vi "disconnect and destroy.vi"(8 "error in (no error)":errorcluster, 11 "hwnd in":u32) -> (0 "error out":errorcluster)   [LabVIEW 2011]
uses:
  user32.dll
panel:
  out "return type 2":u32
  out "return type":u32
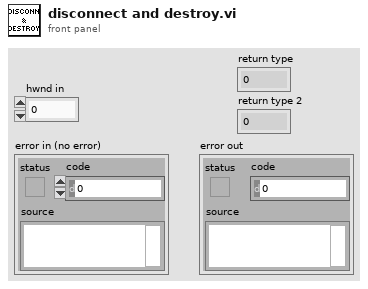
[diagram p1: front panel]
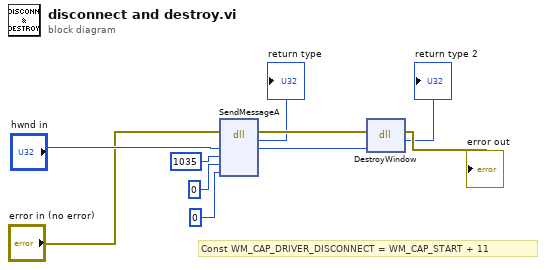
[diagram p0: block diagram]
diagram:
  # "Const WM_CAP_DRIVER_DISCONNECT = WM_CAP_START + 11"
  n1 = dll-call lib="user32.dll" fn="SendMessageA"(error in="error in (no error)", "hwnd"="hwnd in", "msg"=u32 1035, "wParam"=u32 0, "lparam"=u32 0) -> (error out=w8:errorcluster, "return type"=→"return type":u32, "hwnd"=w7:u32)  [unwired: 5 in, 1 out]
  n2 = dll-call lib="user32.dll" fn="DestroyWindow"(error in=w8, "hwnd"=w7) -> (error out=→"error out":errorcluster, "return type"=→"return type 2":u32)  [unwired: 3 in, 1 out]
